vi "ActorDatabase-UpdateReplytoActor.vi"(8 "error in (no error)":errorcluster, 10 "Update Successful":bool, 11 "Database-Actor in":refnum<class "Database-Actor.lvclass">) -> (0 "error out":errorcluster, 3 "Database-Actor out":refnum<class "Database-Actor.lvclass">)   [LabVIEW 2013, in "Database-Actor.lvclass"]
uses:
  Database-Actor.lvclass
  Database-Actor.lvclass/Database-Actor.ctl
  ftw-dataflow/Core/src/JSON/FTW-JSON-RegexParse.vi
  ftw-dataflow/Core/src/Error/FTW-ERR-ThrowGenericError.vi
  ftw-dataflow/Core/src/Container/FTW-Container-Construct.vi
  ftw-dataflow/Core/src/Container/FTW-Container-Load-JSON.vi
  ftw-dataflow/Core/src/Container/FTW-Container-Destroy.vi
  ftw-dataflow/Core/utils/CodeGen/JSON Deserialize/FTW-JSON-Deserialize.xnode
  ITS ERP System/ERP-Container/ERP-ConfigPageNewFeather/ERP-ConfigPageNF.lvclass
  ftw-dataflow/Core/src/Container/FTW-Container.lvclass
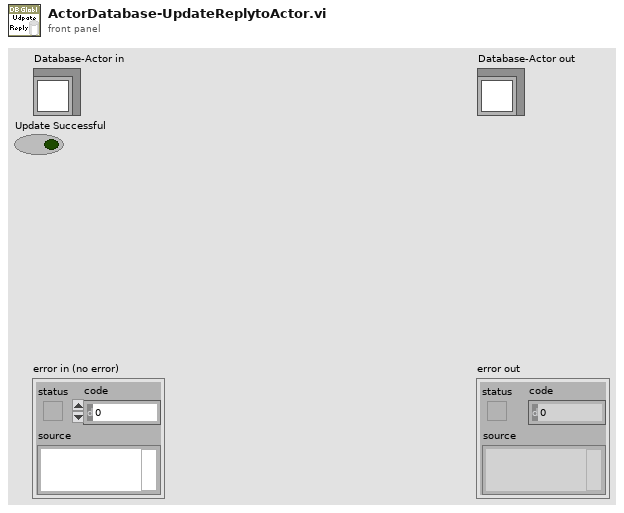
[diagram p1: front panel]
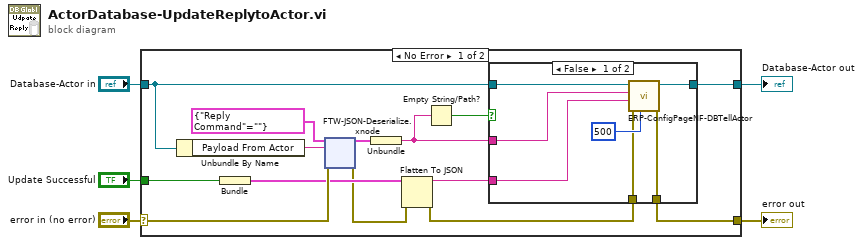
[diagram p0: block diagram]
diagram:
  n1 = case shown="No Error" "error in (no error)" {
    selector: "error in (no error)" -> [w15 w63]
    tunnel: [w13 w63] -> w4
    tunnel: [w18 w62] -> w2
    tunnel: "Database-Actor in" -> [w19 w62]
    tunnel: "Update Successful" -> [w12 _]
    frame No Error {
      n2 = Unbundle By Name(w19) -> ("Payload From Actor"=w16:string)
      n3 = Bundle("Update Successful"=w12) -> (w11:cluster{"Update Successful":bool})  [unwired: 1 in]
      n4 = xnode "FTW-JSON-Deserialize.xnode"("Data Type and Default Values"=cluster{"Reply Command":string} {"Reply Command"=""} ("output cluster"), "JSON String"=w16, "error in"=w15) -> ("Populated Values"=w14:cluster{"Reply Command":string}, "error out"=w10:errorcluster)
      n5 = Unbundle(w14) -> ("Reply Command"=w7:string)
      n6 = Flatten To JSON(anything=w11, error in (no error)=w10) -> (JSON string=w8:string, 11:w9:errorcluster)  [unwired: 1 in]
      n7 = Empty String/Path?(string/path=w7) -> (empty?=w6:bool)
      n8 = case shown="False" w6 {
        tunnel: w19 -> [w25 w28]
        tunnel: [w24 w28] -> w18
        tunnel: [w23 w27] -> w13
        tunnel: w9 -> [w22 w27]
        tunnel: w8 -> [w21 _]
        tunnel: w7 -> [w20 _]
        frame False {
          n9 = call "ERP-ConfigPageNF-DBTellActor.vi"("Timeout"=500, "error in (no error)"=w22, "Message Body"=w21, "Message Header"=w20, "ERP-ConfigPageNF in"=w25) -> ("error out"=w23:errorcluster, "ERP-ConfigPageNF out"=w24:refnum<class "Database-Actor.lvclass">)  [unwired: 4 in, 1 out]
        }
        frame True {
          # "No Reply Needed"
        }
      }
    }
    frame Error {
    }
  }
  "error out" <- w4
  "Database-Actor out" <- w2
